vi "clear Session Data.vi"(0 "OBJ - Measurement Session in":refnum<class "File Session.lvclass">, 11 "error in":errorcluster) -> (4 "OBJ - Measurement Session out":refnum<class "File Session.lvclass">, 15 "error out":errorcluster)   [LabVIEW 2014, in "File Session.lvclass"]
doc: "OVERRIDE VI\nPlaceholder for decendant classes to clear session information and close references."
uses:
  File Session.lvclass
  File Session.lvclass/File Session.ctl
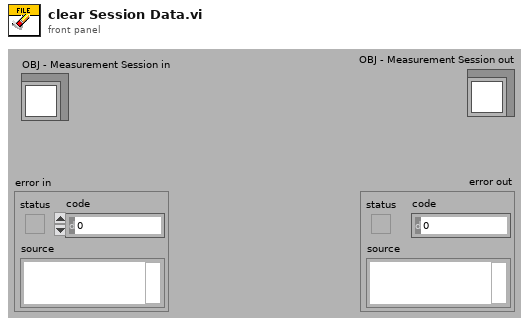
[diagram p1: front panel]
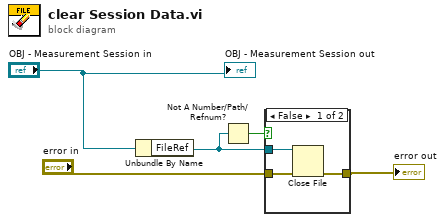
[diagram p0: block diagram]
diagram:
  n1 = Unbundle By Name("OBJ - Measurement Session in") -> ("FileRef"=w5:refnum<file>)
  n2 = Not A Number/Path/Refnum?(number/path/refnum=w5) -> (NaN/Path/Refnum?=w4:bool)
  n3 = case shown="False" w4 {
    tunnel: "error in" -> [w8 w9]
    tunnel: [w7 w9] -> w2
    tunnel: w5 -> [w6 _]
    frame False {
      n4 = Close File(refnum=w6, error in=w8) -> (error out=w7:errorcluster)  [unwired: 1 out]
    }
    frame True {
    }
  }
  "error out" <- w2
  "OBJ - Measurement Session out" <- "OBJ - Measurement Session in"
